vi "Create (dispenser only).vi"(6 "Worktable Mode":T1, 7 "Virtual Mode":bool, 8 "error in":errorcluster, 10 "Config Folder":path=path "C:/Users/husker/Desktop/gantry/Config") -> (0 "error out":errorcluster, 3 "Gantry out":refnum<class "Gantry Class.lvclass">)   [LabVIEW 2011, in "Gantry Class.lvclass"]
uses:
  Gantry Class.lvclass
  WorkTable Class/Type Definitions/Worktable_Mode.ctl
  Gantry Class.lvclass/Gantry Class.ctl
  Config Manager Class/Config Manager Class.lvclass
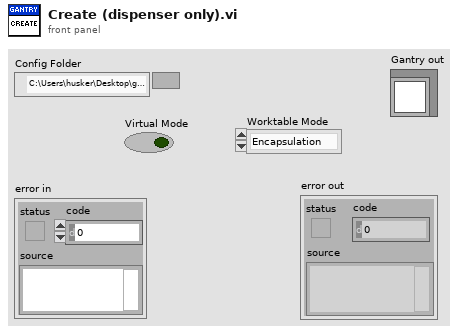
[diagram p1: front panel]
types:
  T1 = typedef "Worktable_Mode.ctl" = enum16{"Encapsulation", "Gluing"}
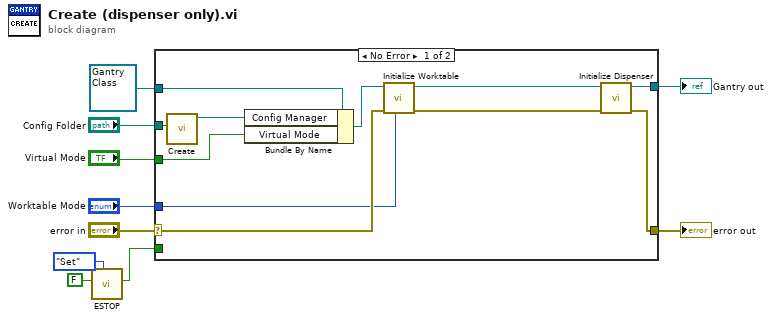
[diagram p0: block diagram]
diagram:
  n1 = call "ESTOP.vi"("Get/Set"=enum16{"Get", "Set"}."Set", "Value In"=FALSE) -> ("Value Out"=w1:bool)  [unwired: 9 in]
  n2 = case shown="No Error" "error in" {
    selector: "error in" -> [w15 w23]
    tunnel: [w20 w23] -> w9
    tunnel: [w21 w22] -> w7
    tunnel: refnum<class "Gantry Class.lvclass"> refnum ("Gantry Class in") -> [w18 w22]
    tunnel: "Config Folder" -> [w17 _]
    tunnel: "Virtual Mode" -> [w19 _]
    tunnel: "Worktable Mode" -> [w13 _]
    tunnel: w1 -> [_ _]
    frame No Error {
      n3 = call "Create.vi"("Config Files Directory"=w17) -> ("Config Manager out"=w16:refnum<class "Config Manager Class.lvclass">)  [unwired: 9 in, 1 out]
      n4 = Bundle By Name(cluster=w18, "Config Manager"=w16, "Virtual Mode"=w19) -> (w14:refnum<class "Gantry Class.lvclass">)
      n5 = call-dynamic "Initialize Worktable.vi"("Worktable Mode"=w13, "error in"=w15, "Gantry in"=w14) -> ("error out"=w11:errorcluster, "Gantry out"=w12:refnum<class "Gantry Class.lvclass">)  [unwired: 7 in]
      n6 = call-dynamic "Initialize Dispenser.vi"("error in"=w11, "Gantry in"=w12) -> ("error out"=w20:errorcluster, "Gantry out"=w21:refnum<class "Gantry Class.lvclass">)  [unwired: 8 in]
    }
    frame Error {
    }
  }
  "error out" <- w9
  "Gantry out" <- w7
